vi "Measure Thermocouple.vi"(6 "ValBufferSize":i32=2048, 7 "MaxTimeMilliseconds":i32 format="%.0g", 8 "error in (no error)":errorcluster {"code" format="%.0x"}, 9 "ChannelList":string, 10 "ThermocoupleType (B)":i32(ring) items=["B", "E", "J", "K", "N", "r", "S", "T"], 11 "instrument handle":refnum<k15>) -> (0 "error out":errorcluster {"code" format="%.0x"}, 1 "ValActualSize":i32, 2 "Val":dbl[](array[numeric]) format="%.2p", 3 "instrument handle out":refnum<k15>)   [LabVIEW 2020, in "Keysight DAQ970.lvlib"]
doc: "Configure the specified channels for Thermocouple Temperature autorange measurements, immediately sweep through the scan list once, and read the measured data. Note: This command redefines the scan list."
uses:
  Keysight DAQ970.lvlib
  KtDAQ970.dll
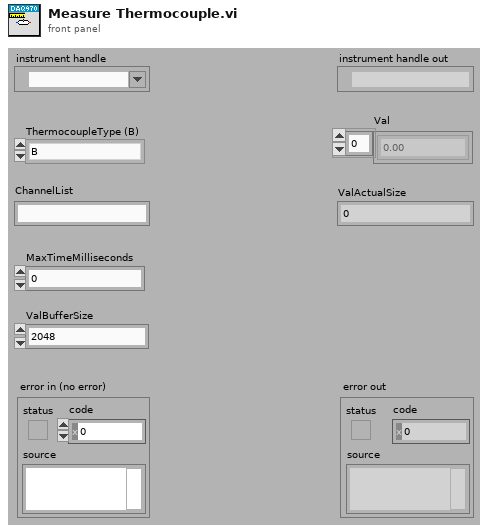
[diagram p1: front panel]
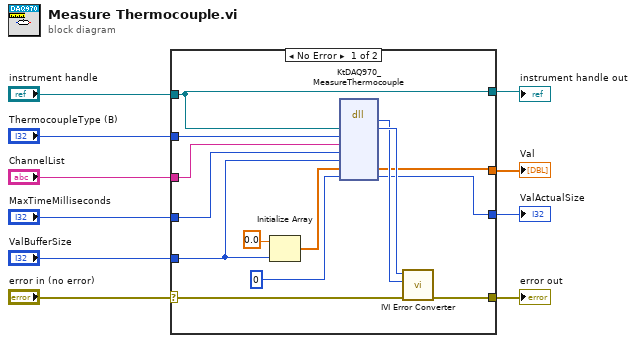
[diagram p0: block diagram]
diagram:
  n1 = case shown="No Error" "error in (no error)" {
    selector: "error in (no error)" -> [w22 w26]
    tunnel: [w21 w26] -> w10
    tunnel: "instrument handle" -> [w12 w25]
    tunnel: "ThermocoupleType (B)" -> [w20 _]
    tunnel: "ChannelList" -> [w19 _]
    tunnel: "MaxTimeMilliseconds" -> [w18 _]
    tunnel: "ValBufferSize" -> [w11 _]
    tunnel: [w15 _] -> w3
    tunnel: [w13 _] -> w2
    tunnel: [w12 w25] -> w1
    frame No Error {
      n2 = Initialize Array(0.0 ("element"), w11) -> (w17:dbl[])
      n3 = dll-call lib="KtDAQ970**.dll" fn="KtDAQ970_MeasureThermocouple"("Vi"=w12, "ThermocoupleType"=w20, "ChannelList"=w19, "MaxTimeMilliseconds"=w18, "ValBufferSize"=w11, "Val"=w17, "ValActualSize"=0) -> (w23:i32, "Vi"=w24:u32, "Val"=w15:dbl[], "ValActualSize"=w13:i32)  [unwired: 7 in, 2 out]
      n4 = call "IVI Error Converter.vi"("error in (no error)"=w22, "IVI error code (0)"=w23, "instrument handle"=w24) -> ("error out"=w21:errorcluster)  [unwired: 7 in, 1 out]
    }
    frame Error {
    }
  }
  "error out" <- w10
  "instrument handle out" <- w1
  "Val" <- w3
  "ValActualSize" <- w2
